vi "MoveToPickupPosition_Lower_Stop.vi"(7 "Lower?":bool, 8 "error in (no error)":errorcluster, 9 "XYZTheta In":dbl[](array[numeric]), 10 "I-O in":refnum<class "I-O.lvclass">, 11 "Motion in":refnum<class "Motion.lvclass">=refnum) -> (0 "error out":errorcluster, 2 "I-O out":refnum<class "I-O.lvclass">, 3 "Motion out":refnum<class "Motion.lvclass">, 5 "Bellow position":dbl[](array[numeric]))   [LabVIEW 2016]
uses:
  Classes/Controller/Motion/Motion Folder/Motion.lvclass
  Classes/Controller/Motion/A3200 Folder/A3200.lvclass
  Classes/Controller/I-O/I-O Folder/I-O.lvclass
  <vilib>/Utility/file.llb/Read Delimited Spreadsheet (DBL).vi
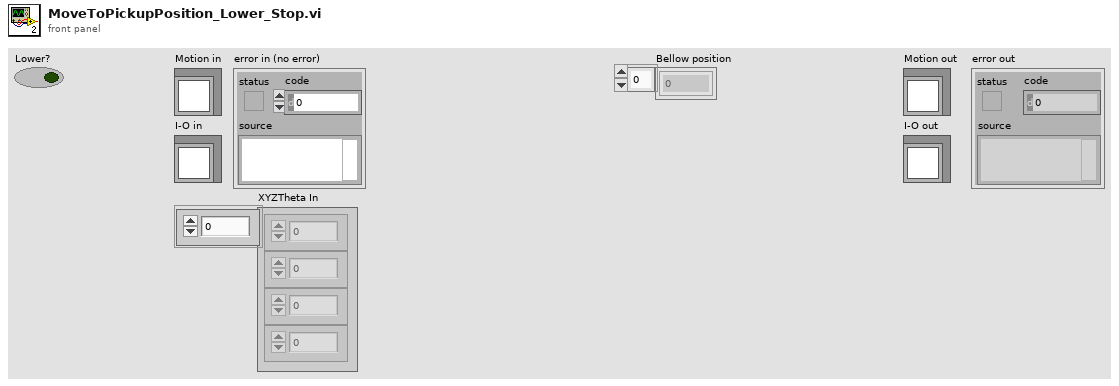
[diagram p1: front panel]
types:
  T1 = typedef "File Paths.ctl" = cluster{"Glue Pattern Folder":path, "Carrier Tray Folder":path, "Pick Up Tool Fixture Folder":path, "Components Folder":path, "Bellows Tool Offset.txt":path, "Pick Up Tool Offset.txt":path, "Dispense Tip Offset.txt":path}
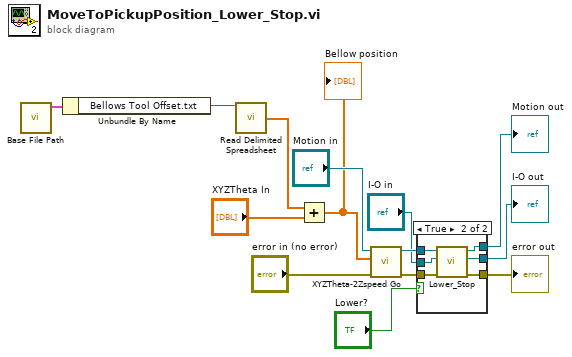
[diagram p0: block diagram]
diagram:
  n1 = call "Base File Path.vi"() -> ("Paths Out"=w8:T1)  [unwired: 11 in]
  n2 = Unbundle By Name(w8) -> ("Bellows Tool Offset.txt"=w7:path)
  n3 = call-poly <vilib>:"Read Delimited Spreadsheet.vi"("file path (dialog if empty)"=w7) -> ("first row"=w6:dbl[])  [unwired: 9 in, 5 out]
  n4 = Add(x=w6, y="XYZTheta In") -> (x+y=w4:dbl[])
  "Bellow position" <- w4
  n5 = call "XYZTheta-2Zspeed Go.vi"("error in (no error)"="error in (no error)", "XYZTheta In"=w4, "Motion in"="Motion in") -> ("error out"=w10:errorcluster, "Motion out"=w13:refnum<class "Motion.lvclass">)  [unwired: 6 in, 1 out]
  n6 = case shown="True" "Lower?" {
    tunnel: w13 -> [w17 w23]
    tunnel: [w17 w22] -> w12
    tunnel: w10 -> [w15 w21]
    tunnel: [w15 w20] -> w9
    tunnel: "I-O in" -> [w16 w19]
    tunnel: [w16 w18] -> w2
    frame False {
    }
    frame True {
      n7 = call "Lower_Stop.vi"("error in (no error)"=w21, "I-O in"=w19, "Motion in"=w23) -> ("error out"=w20:errorcluster, "I-O out"=w18:refnum<class "I-O.lvclass">, "Motion out"=w22:refnum<class "Motion.lvclass">)  [unwired: 6 in]
    }
  }
  "Motion out" <- w12
  "error out" <- w9
  "I-O out" <- w2
